vi "Decrement Survey Point.vi"(0 "Current Point":T1 {"Latitude" format="%#_10g"; "Longitude" format="%#_10g"}, 9 "Bearing":dbl, 11 "Error In":errorcluster) -> (4 "New Point":T1 {"Latitude" format="%#_10g"; "Longitude" format="%#_10g"}, 15 "Error Out":errorcluster)   [LabVIEW 2014]
uses:
  Lat Long Conversion/Controls/PointLatLon.ctl
  Lat Long Conversion/Increment Bearing.vi
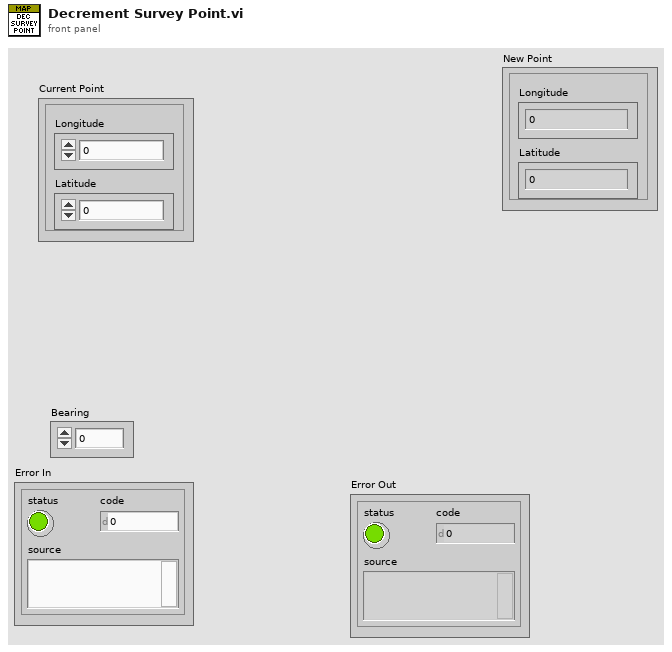
[diagram p1: front panel]
types:
  T1 = typedef "PointLatLon.ctl" = cluster{"Longitude":dbl, "Latitude":dbl}
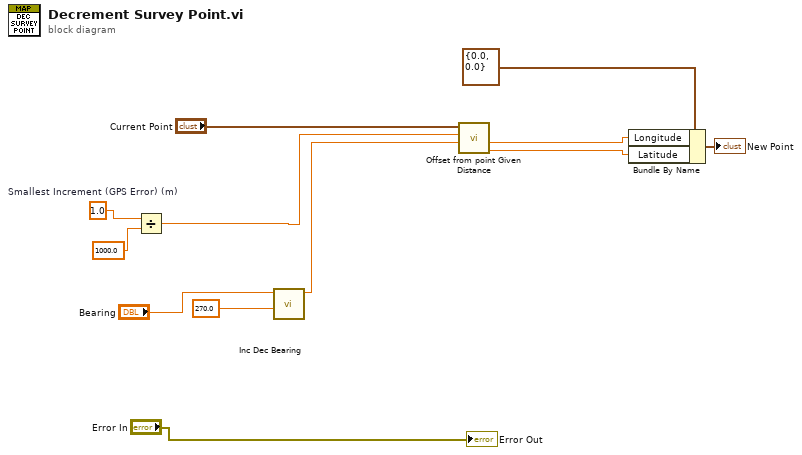
[diagram p0: block diagram]
diagram:
  w2 = 1.0  # Smallest Increment (GPS Error) (m)
  n1 = Divide(x=w2, y=1000.0) -> (x/y=w11:dbl)
  n2 = call-poly "Inc Dec Bearing.vi"("Increment Value"=270.0, "Bearing"="Bearing") -> ("New Bearing"=w8:dbl)  [unwired: 8 in, 1 out]
  n3 = call "Offset from point Given Distance.vi"("Bearing (clockwise from North)"=w8, "Distance (km)"=w11, "Origin Point"="Current Point") -> ("Lat of new point"=w5:dbl, "Lon of new point"=w6:dbl)  [unwired: 5 in, 2 out]
  n4 = Bundle By Name(cluster=T1 {"Longitude"=0.0, "Latitude"=0.0} ("Current Point"), "Longitude"=w6, "Latitude"=w5) -> (→"New Point":T1)
  "Error Out" <- "Error In"
